vi "Execute Query.vi"(4 "error in (no error)":errorcluster, 5 "Return Data? (f)":bool, 6 "Query Name":string, 7 "Statement Refnum":T1) -> (0 "error out":errorcluster, 1 "Data Present?":bool, 2 "Number of Columns":i32, 3 "Statement Refnum":T1)   [LabVIEW 2011]
doc: "Appelle la requête ACCESS et l'éxécute en tenant compte des paramètres chargés"
uses:
  SQL Controls/Statement Refnum.ctl
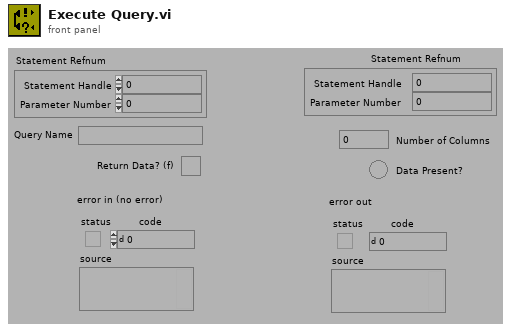
[diagram p1: front panel]
types:
  T1 = typedef "Statement Refnum.ctl" = cluster{"Statement Handle":i32, "Parameter Number":u16}
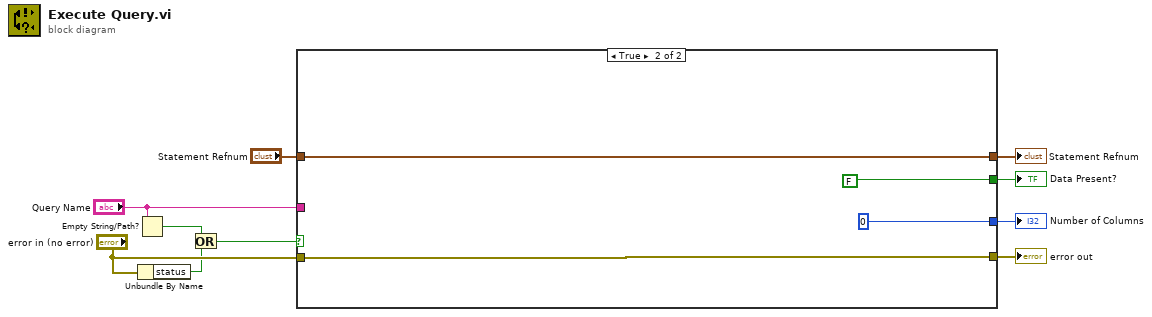
[diagram p0: block diagram]
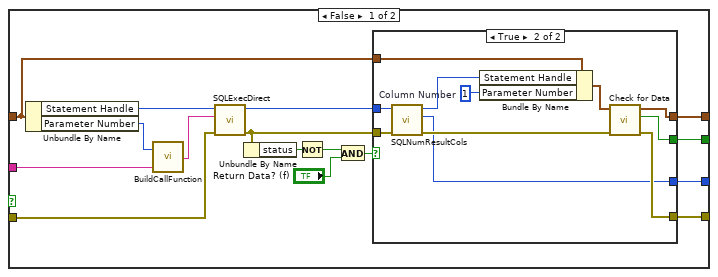
[diagram p2: hidden frame]
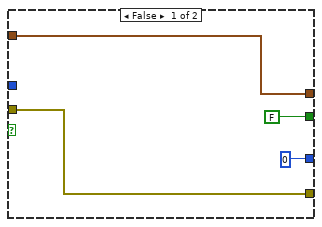
[diagram p3: hidden frame]
diagram:
  n1 = Empty String/Path?(string/path="Query Name") -> (empty?=w3:bool)
  n2 = Unbundle By Name("error in (no error)") -> ("status"=w1:bool)
  n3 = Or(x=w3, y=w1) -> (x .or. y?=w2:bool)
  n4 = case shown="True" w2 {
    tunnel: "Statement Refnum" -> [w14 w45]
    tunnel: [w26 w45] -> w9
    tunnel: [w25 FALSE] -> w8
    tunnel: "error in (no error)" -> [w18 w44]
    tunnel: [w23 w44] -> w6
    tunnel: [w15 0] -> w5
    tunnel: "Query Name" -> [w11 _]
    frame False {
      n5 = Unbundle By Name(w14) -> ("Statement Handle"=w20:i32, "Parameter Number"=w24:u16)
      n6 = call "BuildCallFunction.vi"("StatementName"=w11, "ParameterNum"=w24) -> ("StatementText"=w19:string)
      n7 = call "SQLExecDirect.vi"("error in (no error)"=w18, "StatementText"=w19, "InputHandle"=w20) -> ("error out"=w17:errorcluster, "OutputHandle"=w13:i32)  [unwired: 2 in, 1 out]
      n8 = Unbundle By Name(w17) -> ("status"=w16:bool)
      n9 = Not(x=w16) -> (.not. x?=w12:bool)
      n10 = And(x=w12, y="Return Data? (f)") -> (x .and. y?=w22:bool)
      n11 = case shown="True" w22 {
        tunnel: [w27 w41] -> w26
        tunnel: [FALSE w40] -> w25
        tunnel: [w28 w39] -> w23
        tunnel: w13 -> [_ w38]
        tunnel: w17 -> [w28 w37]
        tunnel: [0 w35] -> w15
        tunnel: w14 -> [w27 w34]
        frame False {
        }
        frame True {
          w32 = u16 1  # Column Number
          n12 = call "SQLNumResultCols.vi"("error in (no error)"=w37, "InputHandle"=w38) -> ("error out"=w36:errorcluster, "NumResultCols"=w35:i32, "OutputHandle"=w31:i32)  [unwired: 3 out]
          n13 = Bundle By Name(cluster=w34, "Statement Handle"=w31, "Parameter Number"=w32) -> (w33:T1)
          n14 = call "Check for Data.vi"("error in (no error)"=w36, "Statement Refnum"=w33) -> ("error out"=w39:errorcluster, "Data Present?"=w40:bool, "Statement Refnum"=w41:T1)  [unwired: 3 out]
        }
      }
    }
    frame True {
    }
  }
  "Statement Refnum" <- w9
  "Data Present?" <- w8
  "error out" <- w6
  "Number of Columns" <- w5
